vi "Untitled 1.vi"() -> ()   [LabVIEW 2016]
uses:
  <vilib>/Utility/miscctls.llb/LVPositionTypeDef.ctl
panel:
  out "Active Row:Active Row Number":i32
  out "Active Row:Active Row Position":T1
  out "Cell BG":u32
  out "Color Box":u32(colorbox)
  out "Selection Color":u32
  out "Listbox 2":i32[](listbox)
  in  "stop":bool
  in  "Listbox":i32[](listbox)
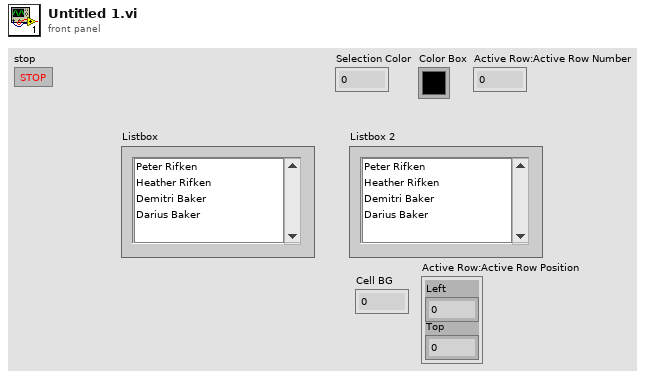
[diagram p1: front panel]
types:
  T1 = typedef "LVPositionTypeDef.ctl" = cluster{"Left":i32, "Top":i32}
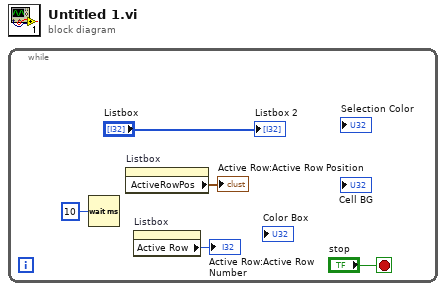
[diagram p0: block diagram]
diagram:
  n1 = while {
    stop <- "stop" stop-if-true
    n2 = Wait (ms)(milliseconds to wait=u32 10) -> ()  [unwired: 1 out]
    n3 = property on="Listbox" class="LstBox (strict)"() -> ("ActiveRowPos"=→"Active Row:Active Row Position":T1)  [unwired: 2 in, 2 out]
    n4 = property on="Listbox" class="LstBox (strict)"() -> ("Active Row"=→"Active Row:Active Row Number":i32)  [unwired: 2 in, 2 out]
    "Listbox 2" <- "Listbox"
  }
